vi "source_target_converter.vi"(0 "Source High":dbl format="%#_13g", 1 "Source Low":dbl format="%#_13g", 2 "Source":dbl[](array[numeric]) format="%#_13g", 3 "Target Low":dbl format="%#_13g", 4 "Target High":dbl format="%#_13g") -> (5 "Target":dbl[](array[numeric]) format="%#_13g")   [LabVIEW 2017, in "sensor_translation.lvlib"]
uses:
  sensor_translation.lvlib
panel:
  out "resulting string":string
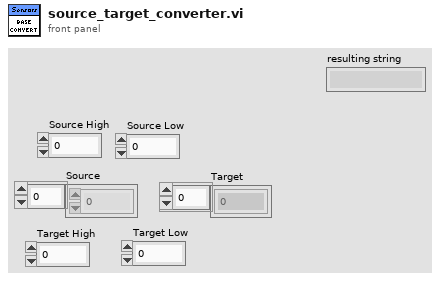
[diagram p1: front panel]
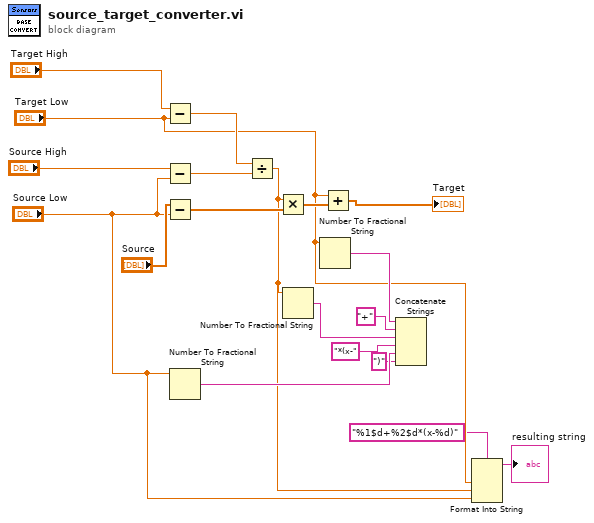
[diagram p0: block diagram]
diagram:
  n1 = Subtract(x="Target High", y="Target Low") -> (x-y=w13:dbl)
  n2 = Subtract(x="Source High", y="Source Low") -> (x-y=w12:dbl)
  n3 = Subtract(x="Source", y="Source Low") -> (x-y=w16:dbl[])
  n4 = Number To Fractional String(number="Source Low") -> (F-format string=w7:string)  [unwired: 3 in]
  n5 = Divide(x=w13, y=w12) -> (x/y=w4:dbl)
  n6 = Multiply(x=w4, y=w16) -> (x*y=w15:dbl[])
  n7 = Number To Fractional String(number=w4) -> (F-format string=w9:string)  [unwired: 3 in]
  n8 = Number To Fractional String(number="Target Low") -> (F-format string=w11:string)  [unwired: 3 in]
  n9 = Add(x="Target Low", y=w15) -> (x+y=→"Target":dbl[])
  n10 = Concatenate Strings(w11, "+" ("string"), w9, "*(x-" ("string"), w7, ")" ("string")) -> ()  [unwired: 1 out]
  n11 = Format Into String(format string="%1$d+%2$d*(x-%d)", "Target Low", w4, "Source Low") -> (resulting string=→"resulting string":string)  [unwired: 2 in, 1 out]
